vi "ProceListActionCase.vi"(9 "DataIn":string, 11 "TypeIn":string) -> (0 "error out":errorcluster)   [LabVIEW 2019]
uses:
  c57c0337-ce4e-4423-b76c-72d0d8df66fc.vi
  29322f98-d6d1-4621-af55-fadb65dc7ba9.vi
  <vilib>/JDP Science/JSONtext/JSON text to Variant.vi
  LLB/Message/MsgShowAndLog.lvlib
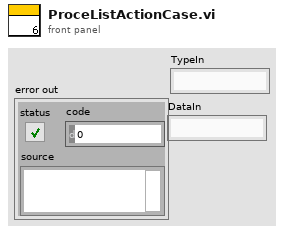
[diagram p1: front panel]
types:
  T1 = enum16{"Initial", "Write", "Read", "Save", "Load", "WrteAll"}
  T2 = enum16{"Initial", "Write", "Read", "Save", "Load", "Add", "Delete"}
  T3 = enum16{"initial", "write", "add", "delete", "Load", "Save", "Read", "ReadProjectName"}
  T4 = cluster{"VirbSeqName":string, "VirbSeqStep":string[]}[]
  T5 = cluster{"VirbSeqName":string, "VirbSeqStep":string[]}
  T6 = cluster{"ProjectName":string, "Parameter":string[][]}
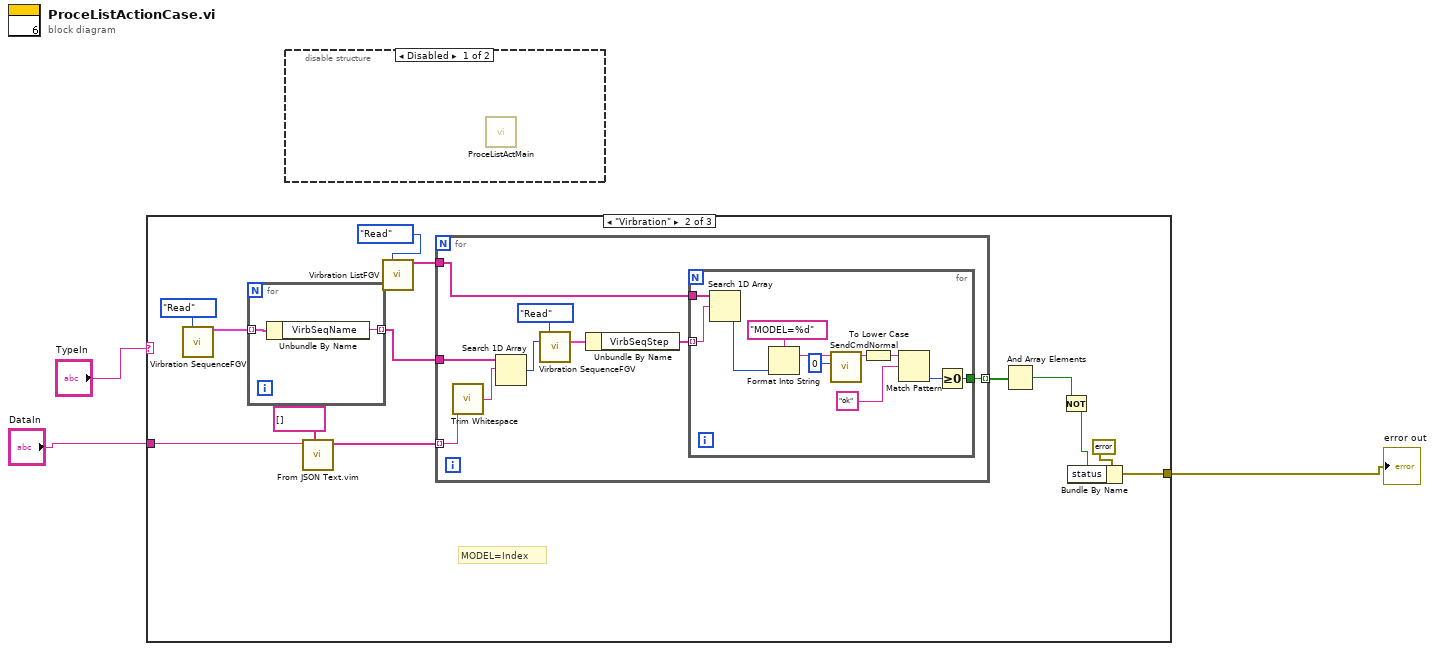
[diagram p0: block diagram]
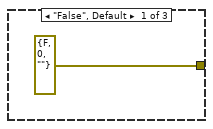
[diagram p3: hidden frame]
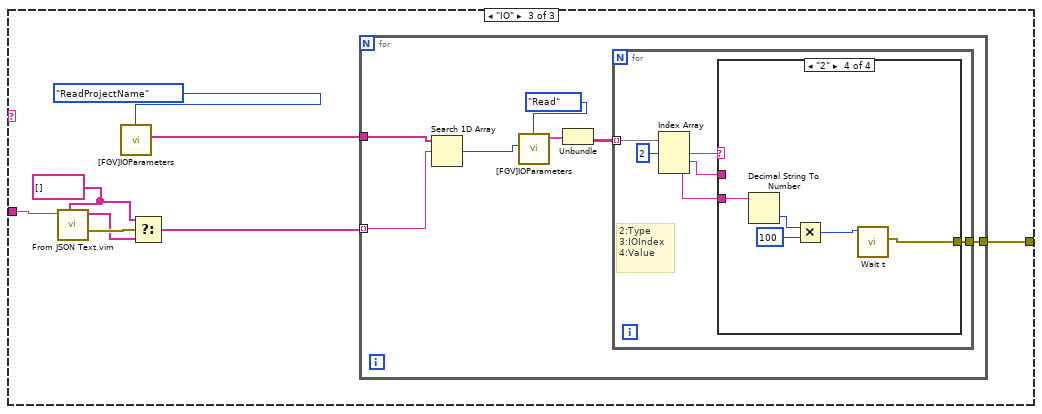
[diagram p4: hidden frame]
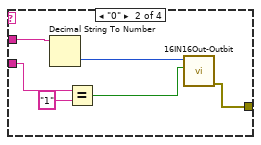
[diagram p6: hidden frame]
diagram:
  n1 = case shown="\"Virbration\"" "TypeIn" {
    tunnel: [errorcluster {"status"=FALSE, "code"=0, "source"=""} ("error out") w13 w40] -> w3
    tunnel: "DataIn" -> [_ w10 w44]
    frame "False", Default {
    }
    frame "Virbration" {
      # "MODEL=Index"
      n2 = call "Virbration SequenceFGV.vi"("Action"=T2."Read") -> ("VirbSeqDataList"=w8:T4)  [unwired: 12 in, 2 out]
      n3 = for {
        tunnel: w8 -> [w19] mode=indexing
        tunnel: [w18] -> w7 mode=indexing
        n4 = Unbundle By Name(w19) -> ("VirbSeqName"=w18:string)
      }
      n5 = call "From JSON Text.vim"("Data Type and Default Value"=string[] [] ("Item Names"), "JSON"=w10) -> ("Data out"=w16:string[])  [unwired: 8 in, 1 out]
      n6 = call "Virbration ListFGV.vi"("Action"=T1."Read") -> ("TableOut"=w5:string[])  [unwired: 12 in, 2 out]
      n7 = for {
        tunnel: w16 -> [w28] mode=indexing
        tunnel: [w26] -> w15 mode=indexing
        tunnel: w7 -> [w25]
        tunnel: w5 -> [w21]
        n8 = call <vilib>:"Trim Whitespace.vi"("string"=w28) -> ("trimmed string"=w27:string)  [unwired: 1 in]
        n9 = Search 1D Array(1D array=w25, element=w27) -> (index of element=w23:i32)  [unwired: 1 in]
        n10 = call "Virbration SequenceFGV.vi"("Action"=T2."Read", "X"=w23) -> ("VirbSeqData"=w22:T5)  [unwired: 11 in, 2 out]
        n11 = Unbundle By Name(w22) -> ("VirbSeqStep"=w20:string[])
        n12 = for {
          tunnel: [w32] -> w26
          tunnel: w21 -> [w31]
          tunnel: w20 -> [w30] mode=indexing
          n13 = Search 1D Array(1D array=w31, element=w30) -> (index of element=w29:i32)  [unwired: 1 in]
          n14 = Format Into String(format string="MODEL=%d", w29) -> (resulting string=w38:string)  [unwired: 2 in, 1 out]
          n15 = call "SendCmdNormal.vi"("index"=0, "DataIn"=w38) -> ("Reccmd"=w36:string)  [unwired: 7 in, 2 out]
          n16 = To Lower Case(string=w36) -> (all lower case string=w34:string)
          n17 = Match Pattern(string=w34, regular expression="ok") -> (offset past match=w33:i32)  [unwired: 1 in, 3 out]
          n18 = Greater Or Equal To 0?(x=w33) -> (x >= 0?=w32:bool)
        }
      }
      n19 = And Array Elements(Boolean array=w15) -> (logical AND=w12:bool)
      n20 = Not(x=w12) -> (.not. x?=w11:bool)
      n21 = Bundle By Name(cluster=errorcluster {"status"=FALSE, "code"=15050, "source"=""} ("error constant"), "status"=w11) -> (w13:errorcluster)
    }
    frame "IO" {
      w46 = string[] [] ("Item Names")
      n22 = call "From JSON Text.vim"("Data Type and Default Value"=w46, "JSON"=w44) -> ("error out"=w47:errorcluster, "Data out"=w45:string[])  [unwired: 8 in]
      n23 = call "[FGV]IOParameters.vi"("Enum"=T3."ReadProjectName") -> ("ProjectName"=w41:string[])  [unwired: 8 in, 2 out]
      n24 = Select(t=w46, s=w47, f=w45) -> (s? t:f=w42:string[])
      n25 = for {
        tunnel: w42 -> [w53] mode=indexing
        tunnel: w41 -> [w54]
        tunnel: [w48] -> w40
        n26 = Search 1D Array(1D array=w54, element=w53) -> (index of element=w51:i32)  [unwired: 1 in]
        n27 = call "[FGV]IOParameters.vi"("Enum"=T3."Read", "ProjectIndex"=w51) -> ("DataOut"=w50:T6)  [unwired: 7 in, 2 out]
        n28 = Unbundle(w50) -> ("Parameter"=w49:string[][])  [unwired: 1 out]
        n29 = for {
          tunnel: w49 -> [w60] mode=indexing
          tunnel: [w55] -> w48
          # "2:Type\n3:IOIndex\n4:Value"
          n30 = Index Array(array=w60, index #1=2 ("index")) -> (element #1=w58:string, element #2=w57:string, element #3=w56:string)  [unwired: 2 in]
          n31 = case shown="\"2\"" w58 {
            tunnel: w57 -> [_ w66 _ _]
            tunnel: w56 -> [_ w64 _ w71]
            tunnel: [_ w61 _ w67] -> w55
            frame "False", Default {
            }
            frame "0" {
              n32 = Decimal String To Number(string=w66) -> (number=w65:i32)  [unwired: 2 in, 1 out]
              n33 = Equal?(x=w64, y="1") -> (x = y?=w62:bool)
              n34 = call "16IN16Out-Outbit.vi"("BL"=w62, "16InOut IO_Output"=w65) -> ("error out"=w61:errorcluster)  [unwired: 9 in]
            }
            frame "1" {
            }
            frame "2" {
              n35 = Decimal String To Number(string=w71) -> (number=w70:i32)  [unwired: 2 in, 1 out]
              n36 = Multiply(x=w70, y=100) -> (x*y=w68:i32)
              n37 = call "Wait t.vi"("wait(ms)"=w68) -> ("error out"=w67:errorcluster)  [unwired: 10 in]
            }
          }
        }
      }
    }
  }
  "error out" <- w3
  n38 = disable-structure shown="Disabled" {
    frame Disabled {
      n39 = call "ProceListActMain.vi"() -> ()  [unwired: 12 in]
    }
    frame Enabled {
    }
  }
